vi "finishPrepareFourthPassPlay.vi"(8 "error in (no error) 2":errorcluster, 10 "Game":refnum<class "Game.lvclass">, 11 "PrepareFourthPassPlay in":refnum<class "PrepareFourthPassPlay.lvclass">) -> (0 "error out 2":errorcluster, 2 "FinishPreparePass?":bool, 3 "PrepareFourthPassPlay out":refnum<class "PrepareFourthPassPlay.lvclass">)   [LabVIEW 2020, in "PrepareFourthPassPlay.lvclass"]
uses:
  PrepareFourthPassPlay.lvclass
  Game_class/Game.lvclass
  Ally_class/Ally.lvclass
  Referee_class/command_interpreted.ctl
  Game_class/Game.lvclass/Game.ctl
  Team_class/Team.lvclass/Team.ctl
  Referee_class/Referee.lvclass/Referee.ctl
  Events_class/Events.lvclass/Events.ctl
  Ally_class/Ally.lvclass/Ally.ctl
  Ally_class/Read PreparePassPlaysEnum.vi
  Ally_class/Write PreparePassPlaysEnum.vi
  Game_class/Read EventsRef.vi
  Events_class/Read ball_out.vi
  Game_class/Read Referee.vi
  Referee_class/Read command_interpreted.vi
  Game_class/Read OffensiveTeam.vi
  Team_class/Read OffensivePlay Finished.vi
  Referee_class/Referee.lvclass
  Events_class/Events.lvclass
panel:
  in  "OffensiveTeam in":refnum<class "Ally.lvclass">
  out "OffensiveTeam out":refnum<class "Ally.lvclass">
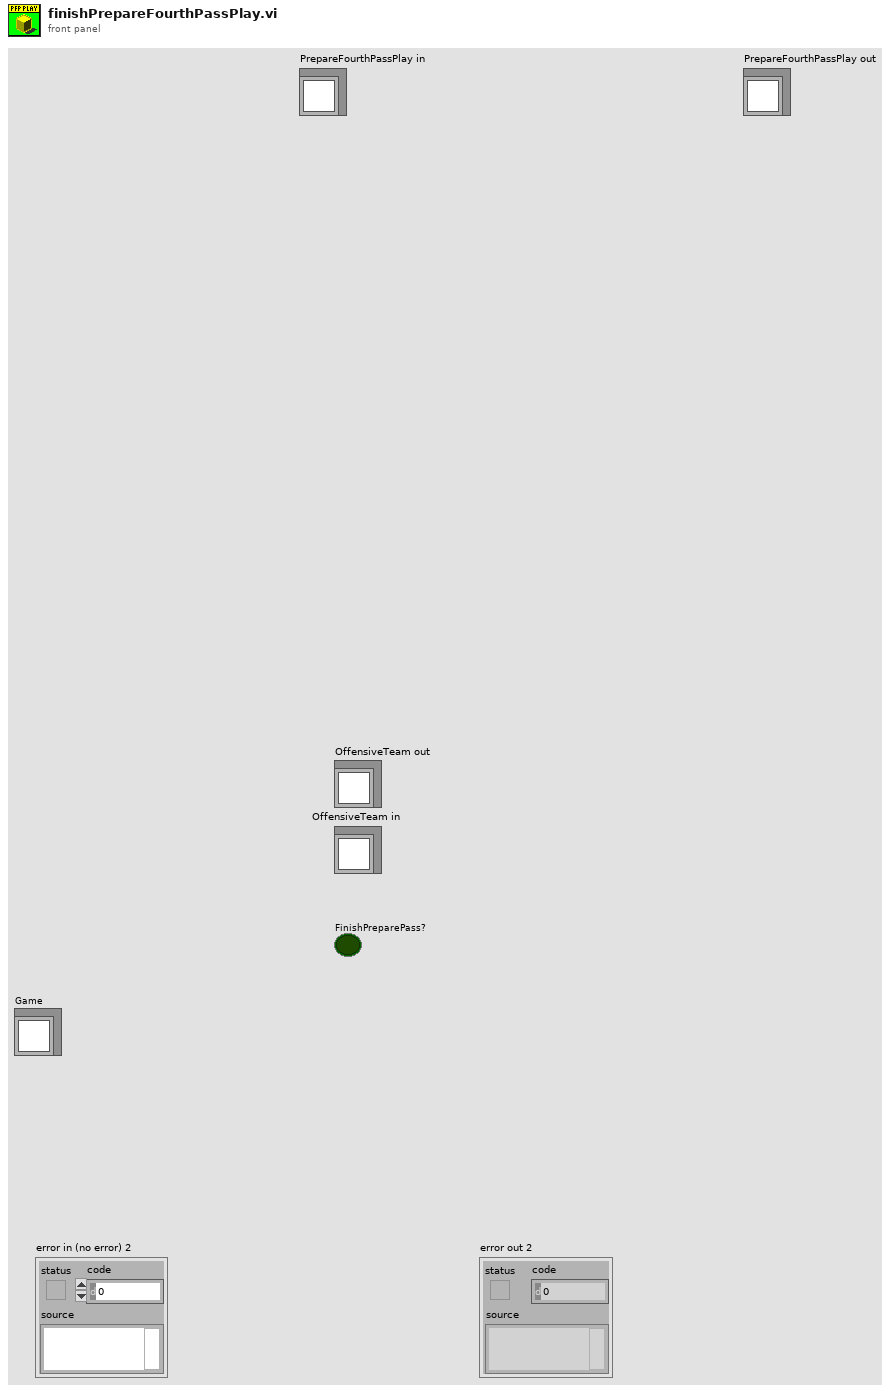
[diagram p1: front panel]
types:
  T1 = typedef "command_interpreted.ctl" = enum16{"Goal Ally", "Goal Enemy", "Ball Placement Enemy", "Ball Placement Ally", "Normal Half Time", "Extra Time  Break", "Extra Half Time", "None", "Post Game", "PKA Normal Start", "Prepare Kickoff Ally", "PKE Normal Start", "Prepare Kickoff Enemy", "Force Start", "Halt", "Timeout", "Prepare Penalty Ally", "Prepare Penalty Enemy", "PPA NormalStart", "PPE Normal Start", "Indirect Free Ally", "Direct Free Enemy", "Direct Free Ally", "Indirect Free Enemy", "Stop"}
  T2 = typedef "OffensivePlay.ctl" = enum16{"PrepareFourthPass", "KeeperPassToStriker", "PrepareKeeperPass", "ACBPass", "ABCPass", "PrepareTriplePass", "TableWithStriker", "TableWith2ndStrikerPlay", "PrepareDoublePass", "PrepareRollToPass", "SimplePass", "PreparePass", "PassToStriker", "BallOutOfField", "PassTo2ndStriker", "StopOffensive", "Prepare Penalty Enemy", "EnemyPossessionAtEnemyField", "EnemyPossesionAtOurField", "TestPlay", "PreparePenaltyAlly", "KickPenaltyAlly", "PrepareKickoffAlly", "PrepareKickoffEnemy", "IndirectEnemy", "DirectEnemy", "PreparePassInGame1", "NormalGame", "DirectKick", "Pass", "Halt", "Timeout", "PassPlay", "PenaltyEnemy"}
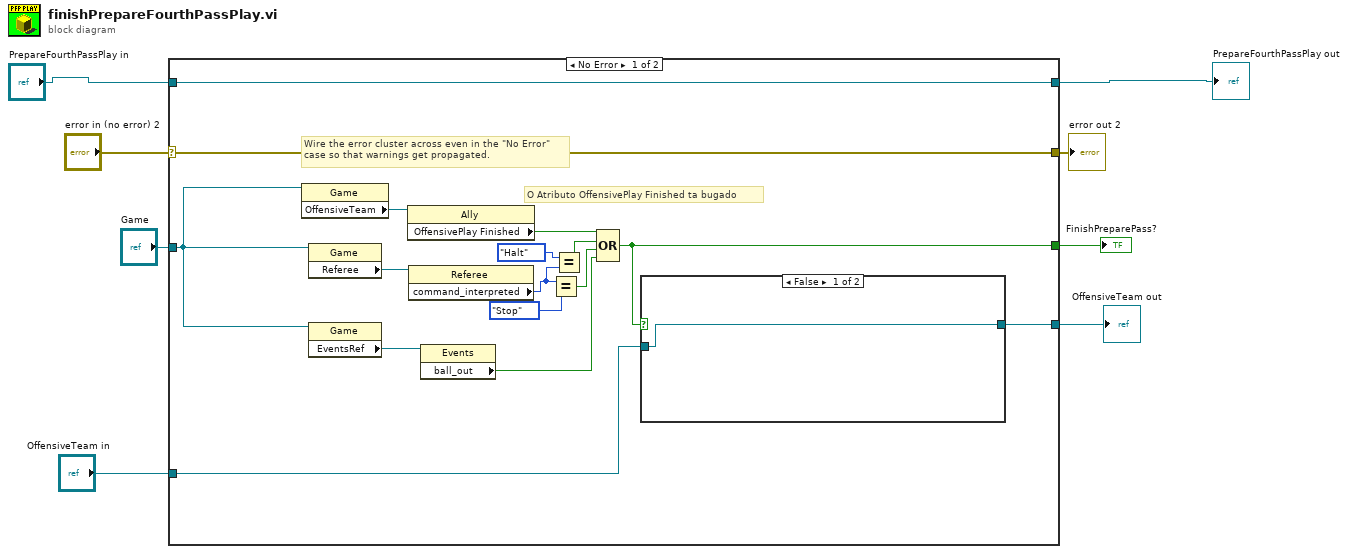
[diagram p0: block diagram]
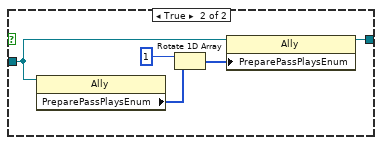
[diagram p2: hidden frame]
diagram:
  n1 = case shown="No Error" "error in (no error) 2" {
    selector: "error in (no error) 2" -> [w23 w32]
    tunnel: [w23 w32] -> w7
    tunnel: [w24 w31] -> w2
    tunnel: "PrepareFourthPassPlay in" -> [w24 w31]
    tunnel: "Game" -> [w20 _]
    tunnel: [w11 _] -> w5
    tunnel: "OffensiveTeam in" -> [w10 _]
    tunnel: [w9 _] -> w3
    frame No Error {
      # "O Atributo OffensivePlay Finished ta bugado"
      # "Wire the error cluster across even in the \"No Error\"\ncase so that warnings get propagated."
      n2 = property class="Game"(reference=w20) -> ("OffensiveTeam"=w22:refnum<class "Ally.lvclass">)  [unwired: 1 in, 2 out]
      n3 = property class="Game"(reference=w20) -> ("Referee"=w21:refnum<class "Referee.lvclass">)  [unwired: 1 in, 2 out]
      n4 = property class="Game"(reference=w20) -> ("EventsRef"=w19:refnum<class "Events.lvclass">)  [unwired: 1 in, 2 out]
      n5 = property class="Ally"(reference=w22) -> ("OffensivePlay Finished"=w12:bool)  [unwired: 1 in, 2 out]
      n6 = property class="Referee"(reference=w21) -> ("command_interpreted"=w16:T1)  [unwired: 1 in, 2 out]
      n7 = property class="Events"(reference=w19) -> ("ball_out"=w13:bool)  [unwired: 1 in, 2 out]
      n8 = Equal?(x=w16, y=command_interpreted."Stop") -> (x = y?=w18:bool)
      n9 = Equal?(x=command_interpreted."Halt" ("y"), y=w16) -> (x = y?=w14:bool)
      n10 = Compound Arithmetic op=OR(w12, w14, w18, w13) -> (w11:bool)
      n11 = case shown="False" w11 {
        tunnel: w10 -> [w25 w27]
        tunnel: [w25 w26] -> w9
        frame False {
        }
        frame True {
          n12 = property class="Ally"(reference=w27) -> ("PreparePassPlaysEnum"=w28:T2[])  [unwired: 1 in, 2 out]
          n13 = Rotate 1D Array(1:w28, 2:1 ("n")) -> (0:w29:T2[])
          n14 = property class="Ally"(reference=w27, "PreparePassPlaysEnum"=w29) -> (reference out=w26:refnum<class "Ally.lvclass">)  [unwired: 1 in, 1 out]
        }
      }
    }
    frame Error {
    }
  }
  "PrepareFourthPassPlay out" <- w2
  "error out 2" <- w7
  "FinishPreparePass?" <- w5
  "OffensiveTeam out" <- w3
